vi "Calculation test.vi"() -> ()   [LabVIEW 2015]
panel:
  in  "Delta Heading":dbl=456.0 format="%#_13g"
  in  "Distance from target":dbl=456.0 format="%#_13g"
  out "Right Of Target":bool
  out "Target Angle":dbl
  out "Target Distance":dbl
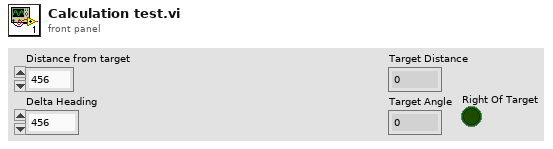
[diagram p1: front panel]
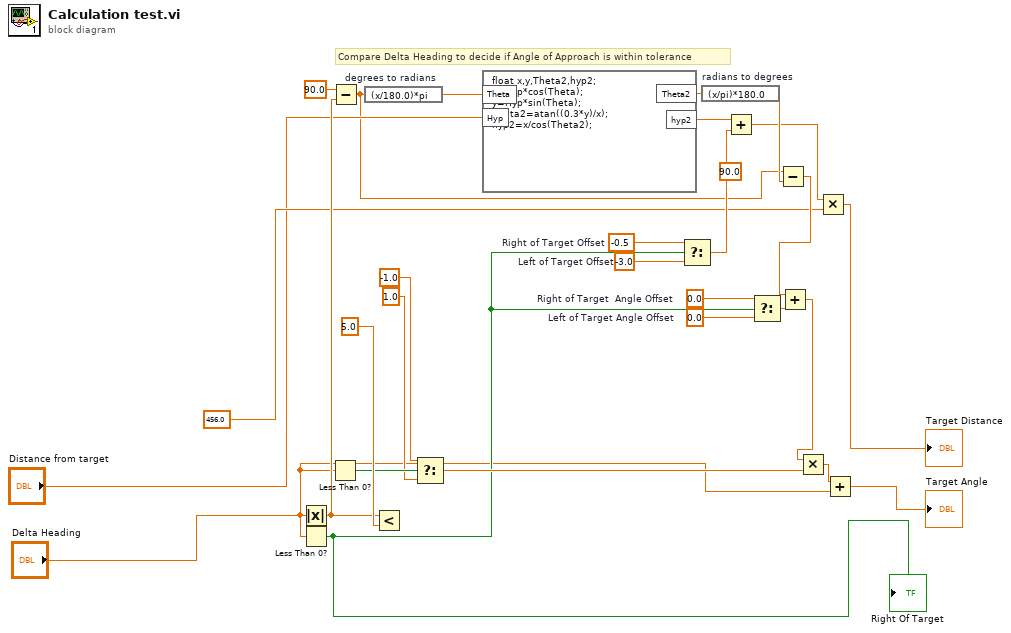
[diagram p0: block diagram]
diagram:
  w7 = 0.0  # Left of Target Angle Offset
  w8 = 0.0  # Right of Target  Angle Offset
  w11 = -3.0  # Left of Target Offset
  w12 = -0.5  # Right of Target Offset
  (unwired) 90.0 ("f")
  # "Compare Delta Heading to decide if Angle of Approach is within tolerance"
  n1 = Absolute Value(x="Delta Heading") -> (abs(x)=w23:dbl)
  n2 = Less Than 0?(x="Delta Heading") -> (x < 0?=w6:bool)
  "Right Of Target" <- w6
  n3 = Less Than 0?(x="Delta Heading") -> (x < 0?=w27:bool)
  n4 = Subtract(x=90.0 ("f"), y=w23) -> (x-y=w1:dbl)
  n5 = expression code="(x/180.0)*pi" "degrees to radians"(w1) -> (w20:dbl)
  n6 = Less?(x=w23, y=5.0) -> ()  [unwired: 1 out]
  n7 = Select(t=-1.0, s=w27, f=1.0) -> (s? t:f=w22:dbl)
  n8 = formula code="float x,y,Theta2,hyp2;\nx=Hyp*cos(Theta);\ny=Hyp*sin(Theta);\nTheta2=atan((0.3*y)/x);\nhyp2=x/cos(Theta2);"("Theta"=w20, "Hyp"="Distance from target") -> ("Theta2"=w19:dbl, "hyp2"=w15:dbl)
  n9 = Select(t=w12, s=w6, f=w11) -> (s? t:f=w13:dbl)
  n10 = expression code="(x/pi)*180.0" "radians to degrees"(w19) -> (w17:dbl)
  n11 = Add(x=w15, y=w13) -> (x+y=w14:dbl)
  n12 = Select(t=w8, s=w6, f=w7) -> (s? t:f=w9:dbl)
  n13 = Subtract(x=w1, y=w17) -> (x-y=w16:dbl)
  n14 = Add(x=w16, y=w9) -> (x+y=w10:dbl)
  n15 = Multiply(x=w10, y=w22) -> (x*y=w21:dbl)
  n16 = Multiply(x=w14, y=456.0 ("Encoder Count Per Calc Ft")) -> (x*y=→"Target Distance":dbl)
  n17 = Add(x=w21, y="Delta Heading") -> (x+y=→"Target Angle":dbl)
